vi "Start.vi"(8 "error in (no error)":errorcluster, 10 "Message in":refnum<class "StartMessage.lvclass">, 11 "DAQMH121119OrcaFlash in":refnum<class "DAQOrcaFlash.lvclass">) -> (0 "error out":errorcluster, 3 "DAQMH121119OrcaFlash out":refnum<class "DAQOrcaFlash.lvclass">)   [LabVIEW 2012, in "DAQOrcaFlash.lvclass"]
doc: "This member function is called when the statemachine in the run.vi receives an 'start' command. It relays the message to all observers of the component.\n\nOverride this member function in your derived class if you need additional start functionality (but don't forget to call the parent method)."
uses:
  DAQOrcaFlash.lvclass
  <vilib>/Distrio/Murmex/StartMessage/StartMessage.lvclass
  <vilib>/Distrio/Murmex/Murmex/Murmex.lvclass
  <vilib>/Distrio/Murmex/ProceedMessage/ProceedMessage.lvclass
  <vilib>/Distrio/Murmex/GenericMessage/GenericMessage.lvclass
  imaging_mode.ctl
  trigger_source.ctl
  trigger_mode.ctl
  DAQOrcaFlash.lvclass/DAQOrcaFlash.ctl
  <vilib>/Distrio/Murmex/Message/Add or replace parameter.vi
  <vilib>/Distrio/Murmex/Message/Message.lvclass
panel:
  # "This method is called when the START\ntrigger is sent. \n\nOverride this method when your component needs to\nrespond to this trigger. \n\nCall parent for proper implementation"
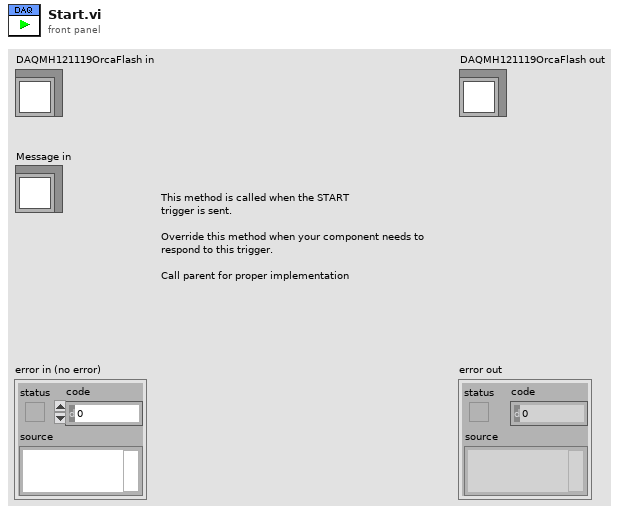
[diagram p1: front panel]
types:
  T1 = typedef "DAQOrcaFlash.lvclass/imaging_mode.ctl" = enum16{"focus mode", "single sweep"}
  T2 = typedef "Murmex.lvlib/StartMessage.lvclass/run mode enum.ctl" = enum16{"infinite", "finite"}
  T3 = typedef "DAQOrcaFlash.lvclass/trigger_mode.ctl" = sgl
  T4 = typedef "DAQOrcaFlash.lvclass/trigger_source.ctl" = sgl
  T5 = cluster{"height":u32, "width":u32, "datatype":u32}
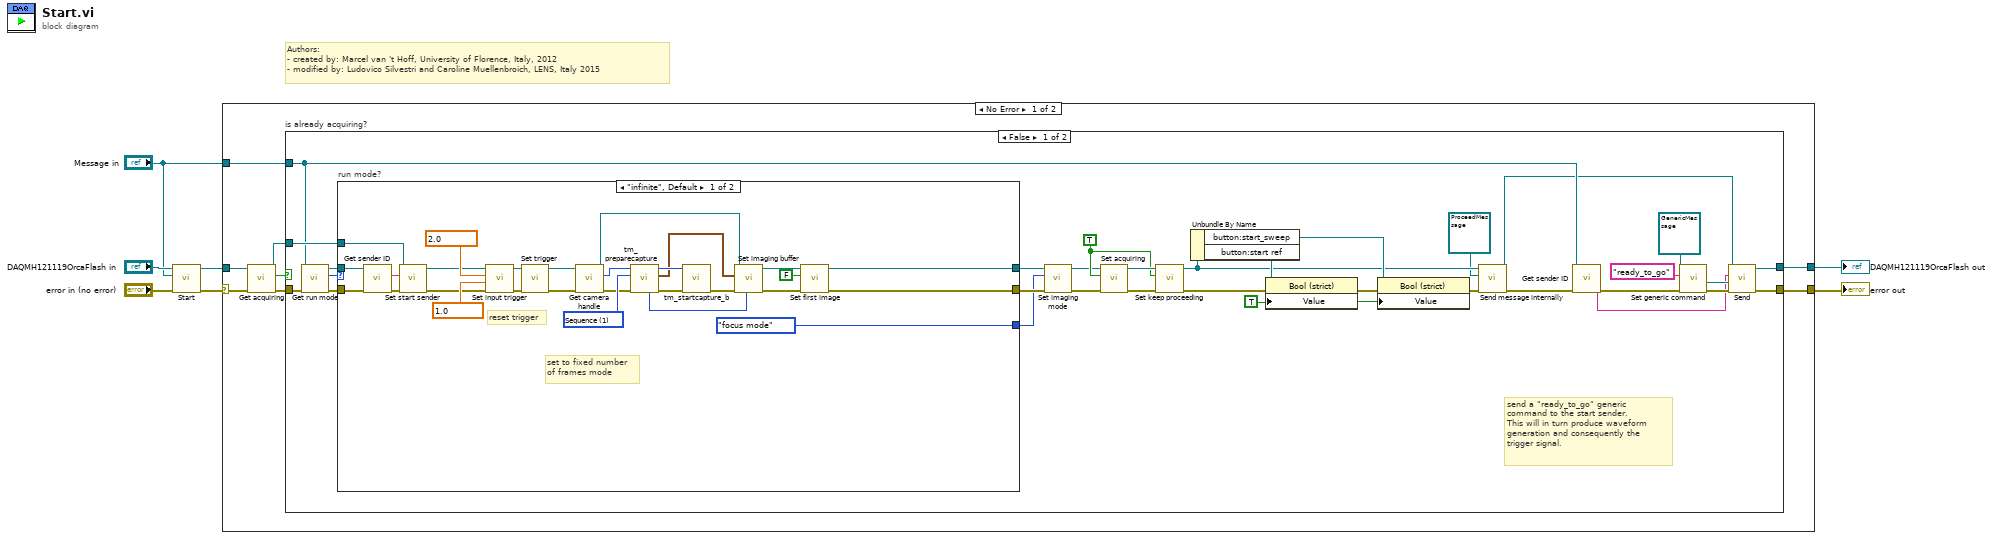
[diagram p0: block diagram]
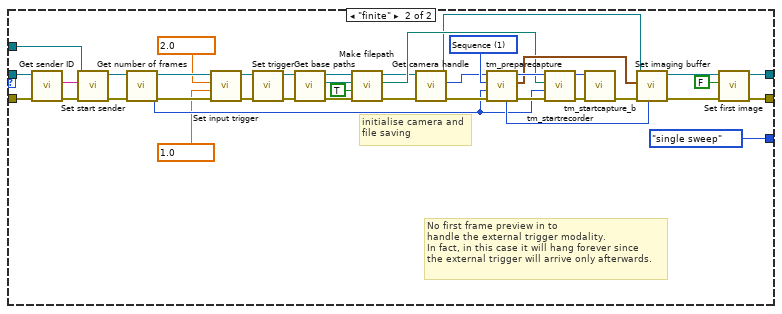
[diagram p2: hidden frame]
diagram:
  # "Authors: \n- created by: Marcel van 't Hoff, University of Florence, Italy, 2012\n- modified by: Ludovico Silvestri and Caroline Muellenbroich, LENS, Italy 2015"
  n1 = call-parent "Start.vi"("error in (no error)"="error in (no error)", "Message in"="Message in", "Murmex in"="DAQMH121119OrcaFlash in") -> ("error out"=w3:errorcluster, "Murmex out"=w4:refnum<class "DAQOrcaFlash.lvclass">)  [unwired: 7 in]
  n2 = case shown="No Error" w3 {
    selector: w3 -> [w9 w119]
    tunnel: [w15 w119] -> w2
    tunnel: [w14 w118] -> w7
    tunnel: w4 -> [w8 w118]
    tunnel: "Message in" -> [w10 _]
    frame No Error {
      n3 = call "Get acquiring.vi"("error in (no error)"=w9, "DAQMH121119OrcaFlash in"=w8) -> ("error out"=w12:errorcluster, "is acquiring?"=w11:bool, "DAQMH121119OrcaFlash out"=w13:refnum<class "DAQOrcaFlash.lvclass">)  [unwired: 7 in]
      n4 = case "is already acquiring?" shown="False" w11 {
        tunnel: [w20 w117] -> w15
        tunnel: [w19 w116] -> w14
        tunnel: w13 -> [w42 w116]
        tunnel: w12 -> [w38 w117]
        tunnel: w10 -> [w25 _]
        frame False {
          w45 = TRUE ("Value")
          w33 = TRUE ("is acquiring?")
          # "send a \"ready_to_go\" generic\ncommand to the start sender.\nThis will in turn produce waveform\ngeneration and consequently the\ntrigger signal."
          n5 = call <vilib>:"Get run mode.vi"("error in (no error)"=w38, "StartMessage in"=w25) -> ("error out"=w37:errorcluster, "run mode"=w36:T2, "StartMessage out"=w35:refnum<class "StartMessage.lvclass">)  [unwired: 7 in]
          n6 = case "run mode?" shown="\"infinite\", Default" w36 {
            tunnel: w37 -> [w61 w100]
            tunnel: [w50 w86] -> w47
            tunnel: [w49 w84] -> w41
            tunnel: w42 -> [w59 w83]
            tunnel: [imaging_mode."focus mode" ("imaging mode") imaging_mode."single sweep" ("imaging mode")] -> w40
            tunnel: w35 -> [w60 w99]
            frame "infinite", Default {
              w64 = T3 1.0 items=["Normal"=1.0, "Start"=6.0] ("Trigger mode")
              w65 = T4 2.0 items=["Internal"=1.0, "External"=2.0, "Software"=3.0] ("Trigger source")
              w73 = 1 items=["Snap", "Sequence"] ("Capture mode")
              # "reset trigger"
              # "set to fixed number\nof frames mode"
              n7 = call <vilib>:"Get sender ID.vi"("error in (no error)"=w61, "Message in"=w60) -> ("error out"=w63:errorcluster, "sender"=w62:string)  [unwired: 7 in, 1 out]
              n8 = call-dynamic "Set start sender.vi"("error in (no error)"=w63, "start sender"=w62, "DAQOrcaFlash in"=w59) -> ("error out"=w48:errorcluster, "DAQOrcaFlash out"=w58:refnum<class "DAQOrcaFlash.lvclass">)  [unwired: 7 in]
              n9 = call-dynamic "Set input trigger.vi"("error in (no error)"=w48, "Trigger mode"=w64, "Trigger source"=w65, "DAQOrcaFlash in"=w58) -> ("error out"=w66:errorcluster, "DAQOrcaFlash out"=w67:refnum<class "DAQOrcaFlash.lvclass">)  [unwired: 6 in]
              n10 = call-dynamic "Set trigger.vi"("error in (no error)"=w66, "DAQOrcaFlash in"=w67) -> ("error out"=w56:errorcluster, "DAQOrcaFlash out"=w57:refnum<class "DAQOrcaFlash.lvclass">)  [unwired: 8 in]
              n11 = call "Get camera handle.vi"("error in (no error)"=w56, "DAQMH121119OrcaFlash in"=w57) -> ("error out"=w68:errorcluster, "cam handle"=w69:u32, "DAQMH121119OrcaFlash out"=w55:refnum<class "DAQOrcaFlash.lvclass">)  [unwired: 7 in]
              n12 = call <userlib>:"tm_preparecapture.vi"("error in (no error)"=w68, "Capture mode"=w73, "Handle in"=w69) -> ("error out"=w74:errorcluster, "Buffer Info"=w71:T5, "Handle out"=w72:u32, "Image type"=w70:u32)  [unwired: 5 in]
              n13 = call <userlib>:"tm_startcapture_b.vi"("error in (no error)"=w74, "Handle in"=w72) -> ("error out"=w54:errorcluster)  [unwired: 8 in, 1 out]
              n14 = call "Set imaging buffer.vi"("Image type"=w70, "error in (no error)"=w54, "Buffer"=w71, "DAQMH121119OrcaFlash in"=w55) -> ("error out"=w51:errorcluster, "DAQMH121119OrcaFlash out"=w52:refnum<class "DAQOrcaFlash.lvclass">)  [unwired: 6 in]
              n15 = call-dynamic "Set first image.vi"("error in (no error)"=w51, "first image acquired?"=FALSE, "DAQOrcaFlash in"=w52) -> ("error out"=w50:errorcluster, "DAQOrcaFlash out"=w49:refnum<class "DAQOrcaFlash.lvclass">)  [unwired: 7 in]
            }
            frame "finite" {
              w79 = T3 1.0 items=["Normal"=1.0, "Start"=6.0] ("Trigger mode")
              w80 = T4 2.0 items=["Internal"=1.0, "External"=2.0, "Software"=3.0] ("Trigger source")
              w113 = 1 items=["Snap", "Sequence"] ("Capture mode")
              # "No first frame preview in to\nhandle the external trigger modality.\nIn fact, in this case it will hang forever since\nthe external trigger will arrive only afterwards."
              # "initialise camera and\nfile saving"
              n16 = call <vilib>:"Get sender ID.vi"("error in (no error)"=w100, "Message in"=w99) -> ("error out"=w82:errorcluster, "sender"=w81:string)  [unwired: 7 in, 1 out]
              n17 = call-dynamic "Set start sender.vi"("error in (no error)"=w82, "start sender"=w81, "DAQOrcaFlash in"=w83) -> ("error out"=w76:errorcluster, "DAQOrcaFlash out"=w77:refnum<class "DAQOrcaFlash.lvclass">)  [unwired: 7 in]
              n18 = call "Get number of frames.vi"("error in (no error)"=w76, "DAQMH121119OrcaFlash in"=w77) -> ("error out"=w93:errorcluster, "no. of frames"=w90:i32, "DAQMH121119OrcaFlash out"=w94:refnum<class "DAQOrcaFlash.lvclass">)  [unwired: 7 in]
              n19 = call-dynamic "Set input trigger.vi"("error in (no error)"=w93, "Trigger mode"=w79, "Trigger source"=w80, "DAQOrcaFlash in"=w94) -> ("error out"=w95:errorcluster, "DAQOrcaFlash out"=w96:refnum<class "DAQOrcaFlash.lvclass">)  [unwired: 6 in]
              n20 = call-dynamic "Set trigger.vi"("error in (no error)"=w95, "DAQOrcaFlash in"=w96) -> ("error out"=w98:errorcluster, "DAQOrcaFlash out"=w97:refnum<class "DAQOrcaFlash.lvclass">)  [unwired: 8 in]
              n21 = call-dynamic "Get base paths.vi"("error in (no error)"=w98, "DAQOrcaFlash in"=w97) -> ("error out"=w109:errorcluster, "filepath"=w107:path, "DAQOrcaFlash out"=w108:refnum<class "DAQOrcaFlash.lvclass">)  [unwired: 6 in, 1 out]
              n22 = call "Make filepath.vi"("error in (no error)"=w109, "is cxd file path?"=TRUE, "base path"=w107, "DAQOrcaFlash in"=w108) -> ("error out"=w91:errorcluster, "filepath out"=w106:path, "DAQOrcaFlash out"=w92:refnum<class "DAQOrcaFlash.lvclass">)  [unwired: 5 in]
              n23 = call "Get camera handle.vi"("error in (no error)"=w91, "DAQMH121119OrcaFlash in"=w92) -> ("error out"=w102:errorcluster, "cam handle"=w103:u32, "DAQMH121119OrcaFlash out"=w88:refnum<class "DAQOrcaFlash.lvclass">)  [unwired: 7 in]
              n24 = call <userlib>:"tm_preparecapture.vi"("error in (no error)"=w102, "Frames"=w90, "Capture mode"=w113, "Handle in"=w103) -> ("error out"=w114:errorcluster, "Buffer Info"=w110:T5, "Handle out"=w115:u32, "Image type"=w111:u32)  [unwired: 4 in]
              n25 = call <userlib>:"tm_startrecorder.vi"("error in (no error)"=w114, "frames"=w90, "File"=w106, "Handle in"=w115) -> ("error out"=w104:errorcluster, "Handle out"=w105:u32)  [unwired: 6 in]
              n26 = call <userlib>:"tm_startcapture_b.vi"("error in (no error)"=w104, "Handle in"=w105) -> ("error out"=w89:errorcluster)  [unwired: 8 in, 1 out]
              n27 = call "Set imaging buffer.vi"("Image type"=w111, "error in (no error)"=w89, "Buffer"=w110, "DAQMH121119OrcaFlash in"=w88) -> ("error out"=w87:errorcluster, "DAQMH121119OrcaFlash out"=w85:refnum<class "DAQOrcaFlash.lvclass">)  [unwired: 6 in]
              n28 = call-dynamic "Set first image.vi"("error in (no error)"=w87, "first image acquired?"=FALSE, "DAQOrcaFlash in"=w85) -> ("error out"=w86:errorcluster, "DAQOrcaFlash out"=w84:refnum<class "DAQOrcaFlash.lvclass">)  [unwired: 7 in]
            }
          }
          n29 = call "Set imaging mode.vi"("error in (no error)"=w47, "imaging mode"=w40, "DAQMH121119OrcaFlash in"=w41) -> ("error out"=w31:errorcluster, "DAQMH121119OrcaFlash out"=w32:refnum<class "DAQOrcaFlash.lvclass">)  [unwired: 7 in]
          n30 = call "Set acquiring.vi"("error in (no error)"=w31, "is acquiring?"=w33, "DAQMH121119OrcaFlash in"=w32) -> ("error out"=w39:errorcluster, "DAQMH121119OrcaFlash out"=w34:refnum<class "DAQOrcaFlash.lvclass">)  [unwired: 7 in]
          n31 = call-dynamic "Set keep proceeding.vi"("error in (no error)"=w39, "keep proceeding?"=w33, "DAQOrcaFlash in"=w34) -> ("error out"=w30:errorcluster, "DAQOrcaFlash out"=w29:refnum<class "DAQOrcaFlash.lvclass">)  [unwired: 7 in]
          n32 = Unbundle By Name(w29) -> ("button:start_sweep"=w43:refnum<vi>, "button:start ref"=w46:refnum<vi>)
          n33 = property class="Bool (strict)"(reference=w46, error in=w30, "Value"=w45) -> (error out=w44:errorcluster)  [unwired: 1 out]
          n34 = property class="Bool (strict)"(reference=w43, error in=w44, "Value"=w45) -> (error out=w28:errorcluster)  [unwired: 1 out]
          n35 = call <vilib>:"Send message internally.vi"("error in (no error)"=w28, "Message"=refnum<class "ProceedMessage.lvclass"> refnum ("ProceedMessage"), "Murmex in"=w29) -> ("error out"=w26:errorcluster, "Murmex out"=w16:refnum<class "DAQOrcaFlash.lvclass">)  [unwired: 7 in]
          n36 = call <vilib>:"Get sender ID.vi"("error in (no error)"=w26, "Message in"=w25) -> ("error out"=w18:errorcluster, "sender"=w17:string)  [unwired: 7 in, 1 out]
          n37 = call <vilib>:"Set generic command.vi"("error in (no error)"=w18, "generic command"="ready_to_go", "GenericMessage in"=refnum<class "GenericMessage.lvclass"> refnum ("Distrio Murmex 1.5:GenericMessage")) -> ("error out"=w21:errorcluster, "GenericMessage out"=w24:refnum<class "GenericMessage.lvclass">)  [unwired: 7 in]
          n38 = call <vilib>:"Send.vi"("error in (no error)"=w21, "Message"=w24, "recipient"=w17, "Murmex in"=w16) -> ("error out"=w20:errorcluster, "Murmex out"=w19:refnum<class "DAQOrcaFlash.lvclass">)  [unwired: 6 in]
        }
        frame True {
          # "Skip double start trigger events"
        }
      }
    }
    frame Error {
    }
  }
  "DAQMH121119OrcaFlash out" <- w7
  "error out" <- w2
